vi "TEST.vi"() -> ()   [LabVIEW 2012, in "GPP.lvlib"]
uses:
  GPP.lvlib
panel:
  out "Time Used":dbl
  out "Actual Voltage Level (V)":dbl format="%.3f"
  in  "Channel  (1: CH1)":u16(ring)=1 items=["CH1"=1, "CH2"=2, "CH3"=3, "CH4"=4]
  in  "VISA resource name":refnum<visa-resource-name>
  in  "ID Query (True)":bool=TRUE
  in  "Reset (True)":bool=TRUE
  in  "SerialSetting":T1={"Baud Rate"=115200, "Data Bits"=8, "Parity"=0, "Stop Bits"=10} {"Stop Bits" items=["1.0"=10, "1.5"=15, "2.0"=20]; "Parity" items=["None", "Odd", "Even", "Mark", "Space"]}
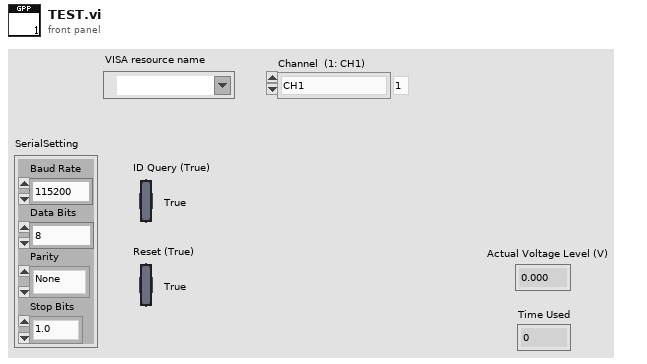
[diagram p1: front panel]
types:
  T1 = cluster{"Baud Rate":u32, "Data Bits":u16, "Parity":u16, "Stop Bits":u16}
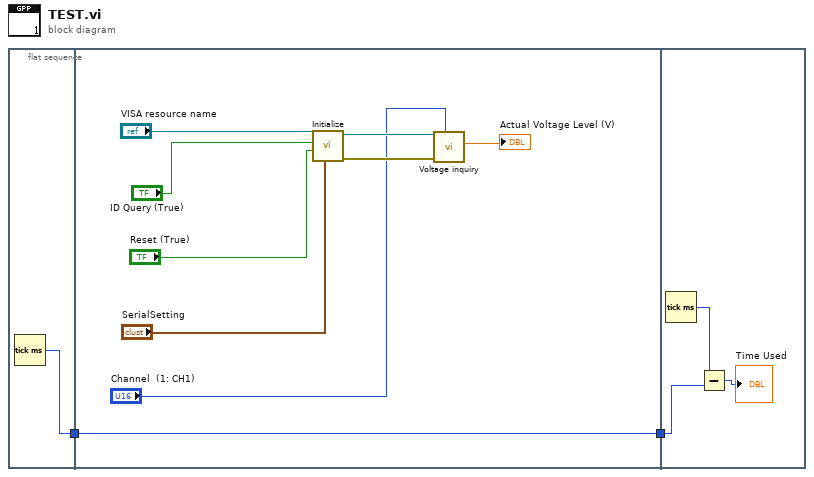
[diagram p0: block diagram]
diagram:
  n1 = flat-sequence {
    tunnel: [w3] -> w1
    tunnel: [w4] -> w2
    tunnel: w1 -> [w4]
    tunnel: w2 -> [w14]
    frame #0 {
      n2 = Tick Count (ms)() -> (millisecond timer value=w3:u32)
    }
    frame #1 {
      n3 = call "Initialize.vi"("SerialSetting"="SerialSetting", "Reset (True)"="Reset (True)", "ID Query (True)"="ID Query (True)", "VISA resource name"="VISA resource name") -> ("error out"=w8:errorcluster, "VISA resource name out"=w7:refnum<visa-resource-name>)  [unwired: 5 in, 1 out]
      n4 = call "Voltage inquiry.vi"("Channel  (1: CH1)"="Channel  (1: CH1)", "error in (no error)"=w8, "VISA resource name"=w7) -> ("Voltage"=→"Actual Voltage Level (V)":dbl)  [unwired: 6 in, 2 out]
    }
    frame #2 {
      n5 = Tick Count (ms)() -> (millisecond timer value=w15:u32)
      n6 = Subtract(x=w15, y=w14) -> (x-y=→"Time Used":u32)
    }
  }
